vi "test.vi"() -> ()   [LabVIEW 2023]
uses:
  Configure.ctl
  36802af5-5fdb-4f05-a304-f04dc6a9e58e.vi
  Aim TTi 1908P DMM.lvlib
  5743e2c1-0597-492e-89b6-aaa377a6e37c.vi
panel:
  out "x-y":dbl[](array[numeric])
  in  "Configuration 2":T1
  in  "error in":errorcluster
  out "read buffer":string[](array[string])
  out "error out":errorcluster
  in  "VISA resource name":refnum<visa-resource-name>
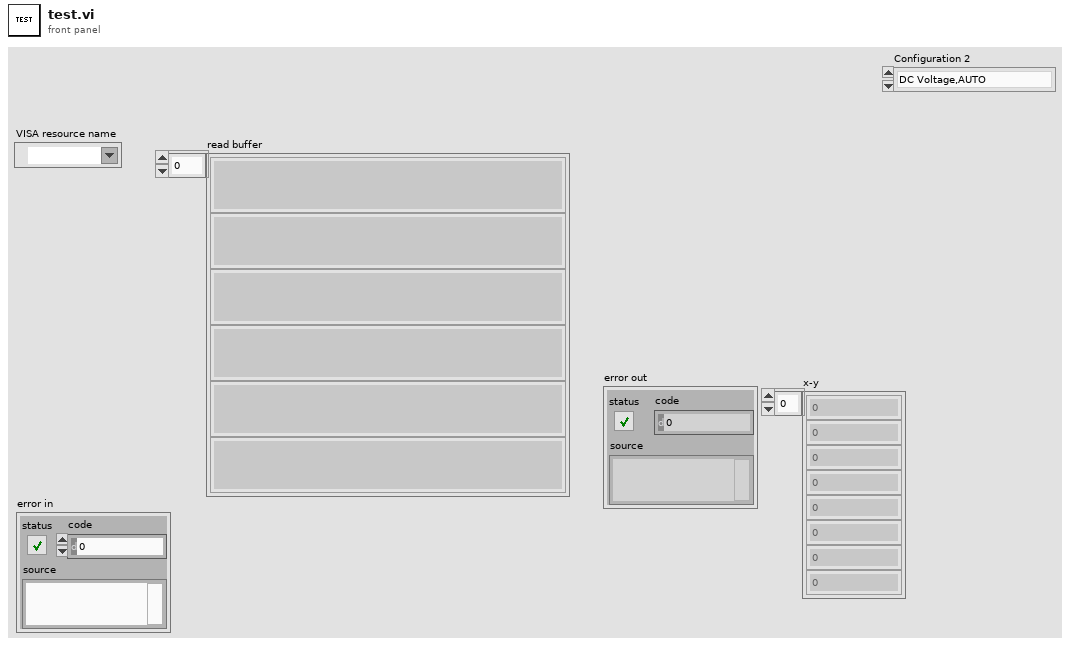
[diagram p1: front panel]
types:
  T1 = typedef "Configure.ctl" = enum16{"DC Voltage,AUTO", "DC Voltage,10V", "Resistance,AUTO", "Resistance,10K"}
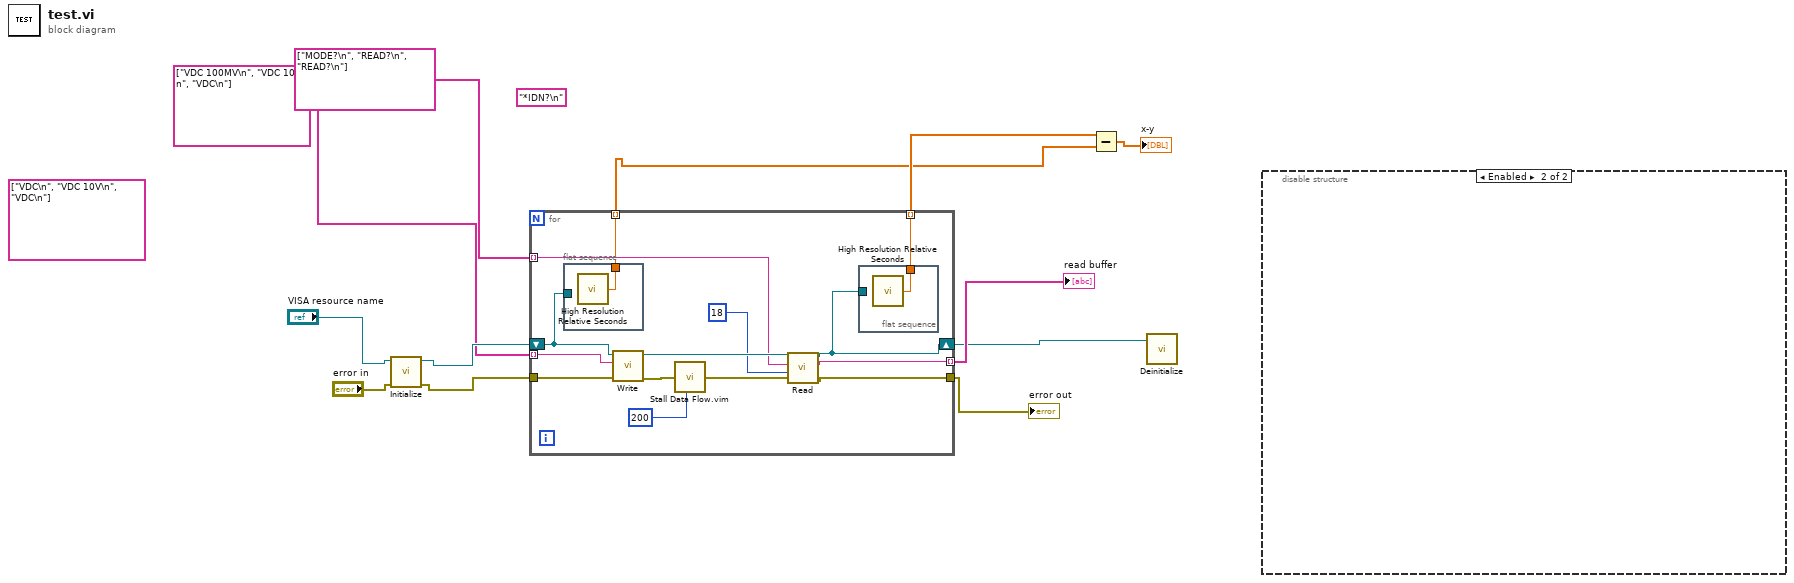
[diagram p0: block diagram]
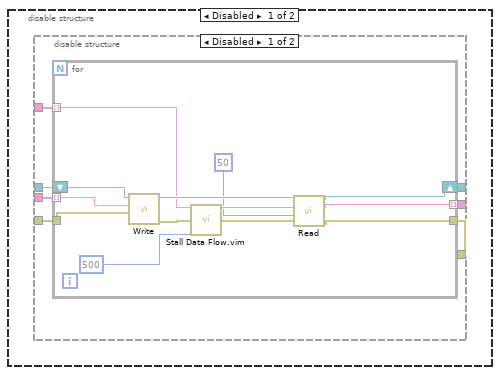
[diagram p2: hidden frame]
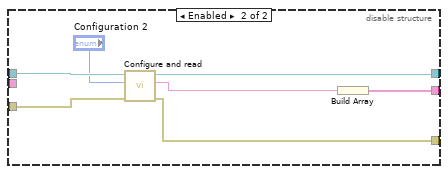
[diagram p3: hidden frame]
diagram:
  (unwired) string[] ["VDC\n", "VDC 10V\n", "VDC\n"] ("write buffer")
  (unwired) "*IDN?\n" ("write buffer")
  n1 = call "Initialize.vi"("error in"="error in", "NI MAX name"="VISA resource name") -> ("error out"=w7:errorcluster, "VISA resource name out"=w8:refnum<visa-resource-name>)  [unwired: 6 in]
  n2 = for {
    tunnel: string[] ["MODE?\n", "READ?\n", "READ?\n"] ("write buffer") -> [w20] mode=indexing
    tunnel: [w24] -> w11 mode=indexing
    tunnel: string[] ["VDC 100MV\n", "VDC 10V\n", "VDC\n"] ("write buffer") -> [w21] mode=indexing
    shift-right: [w17] -> w10
    shift-left: w8 -> [w18]
    tunnel: w7 -> [w23]
    tunnel: [w25] -> w12
    tunnel: [w16] -> w5 mode=indexing
    tunnel: [w15] -> w4 mode=indexing
    n3 = flat-sequence {
      tunnel: w18 -> [_]
      tunnel: [w27] -> w15
      frame #0 {
        n4 = call <vilib>:"High Resolution Relative Seconds.vi"() -> ("relative seconds"=w27:dbl)
      }
    }
    n5 = call "Write.vi"("error in"=w23, "Data to write"=w21, "VISA resource name"=w18) -> ("error out"=w13:errorcluster, "VISA resource name out"=w22:refnum<visa-resource-name>)  [unwired: 5 in]
    n6 = call "Stall Data Flow.vim"("value in"=w13, "milliseconds to wait"=u32 200) -> ("value out"=w26:errorcluster)  [unwired: 1 out]
    n7 = call "Read.vi"("error in"=w26, "byte count"=u32 18, "Read command"=w20, "VISA resource name"=w22) -> ("error out"=w25:errorcluster, "Read data"=w24:string, "VISA resource name out"=w17:refnum<visa-resource-name>)  [unwired: 3 in]
    n8 = flat-sequence {
      tunnel: w17 -> [_]
      tunnel: [w28] -> w16
      frame #0 {
        n9 = call <vilib>:"High Resolution Relative Seconds.vi"() -> ("relative seconds"=w28:dbl)
      }
    }
  }
  "error out" <- w12
  "read buffer" <- w11
  n10 = Subtract(x=w5, y=w4) -> (x-y=→"x-y":dbl[])
  n11 = call "Deinitialize.vi"("VISA resource name"=w10) -> ()  [unwired: 8 in, 1 out]
  n12 = disable-structure shown="Enabled" {
    frame Disabled {
      n13 = disable-structure shown="Disabled" {
        disable-tunnel: _ -> [w35 _]
        disable-tunnel: [w34 w51] -> _
        disable-tunnel: [w33 w48] -> _
        disable-tunnel: _ -> [w32 _]
        disable-tunnel: [w31 w49] -> _
        disable-tunnel: _ -> [w30 w54]
        disable-tunnel: _ -> [w29 w52]
        frame Disabled {
          n14 = for {
            tunnel: w35 -> [w37] mode=indexing
            tunnel: [w43] -> w33 mode=indexing
            tunnel: w32 -> [w38] mode=indexing
            shift-right: [w42] -> w31
            shift-left: w30 -> [w40]
            tunnel: w29 -> [w41]
            tunnel: [w44] -> w34
            n15 = call "Write.vi"("error in"=w41, "Data to write"=w38, "VISA resource name"=w40) -> ("error out"=w46:errorcluster, "VISA resource name out"=w39:refnum<visa-resource-name>)  [unwired: 5 in]
            n16 = call "Stall Data Flow.vim"("value in"=w46, "milliseconds to wait"=u32 500) -> ("value out"=w45:errorcluster)  [unwired: 1 out]
            n17 = call "Read.vi"("error in"=w45, "byte count"=u32 50, "Read command"=w37, "VISA resource name"=w39) -> ("error out"=w44:errorcluster, "Read data"=w43:string, "VISA resource name out"=w42:refnum<visa-resource-name>)  [unwired: 3 in]
          }
        }
        frame Enabled {
          n18 = call "Configure and read.vi"("error in"=w52, "Configuration"="Configuration 2", "VISA resource name"=w54) -> ("error out"=w51:errorcluster, "Read value"=w50:string, "VISA resource name out"=w49:refnum<visa-resource-name>)  [unwired: 4 in]
          n19 = Build Array(w50) -> (w48:string[])
        }
      }
    }
    frame Enabled {
    }
  }
